vi "Read_EPICS_Client_PVs(DataSocket)DBL_20160318.vi"(7 "error in (no error)":errorcluster, 10 "PV name":string="SR-RF2-H2O-VBL:HeatLoad-SBP-HOM") -> (0 "error out 2":errorcluster, 2 "Value(String)":string, 3 "Value":dbl=588.4805608779573, 4 "quality":u64)   [LabVIEW 2013]
panel:
  out "values":T1
  out "found":bool
  out "replaced":bool
  out "variant out":variant
  out "data 3":bool
  out "Value 2":dbl=588.4805608779573
  out "data 2":string
  out "string":i16[](array[numeric])
  out "data string 4":string
  out "type string 2":i16[](array[numeric])
  out "data string 3":string
  out "data":variant
  in  "stop":bool
  out "loop":i32
  # "有@表示為數字"
  # "4\n10"
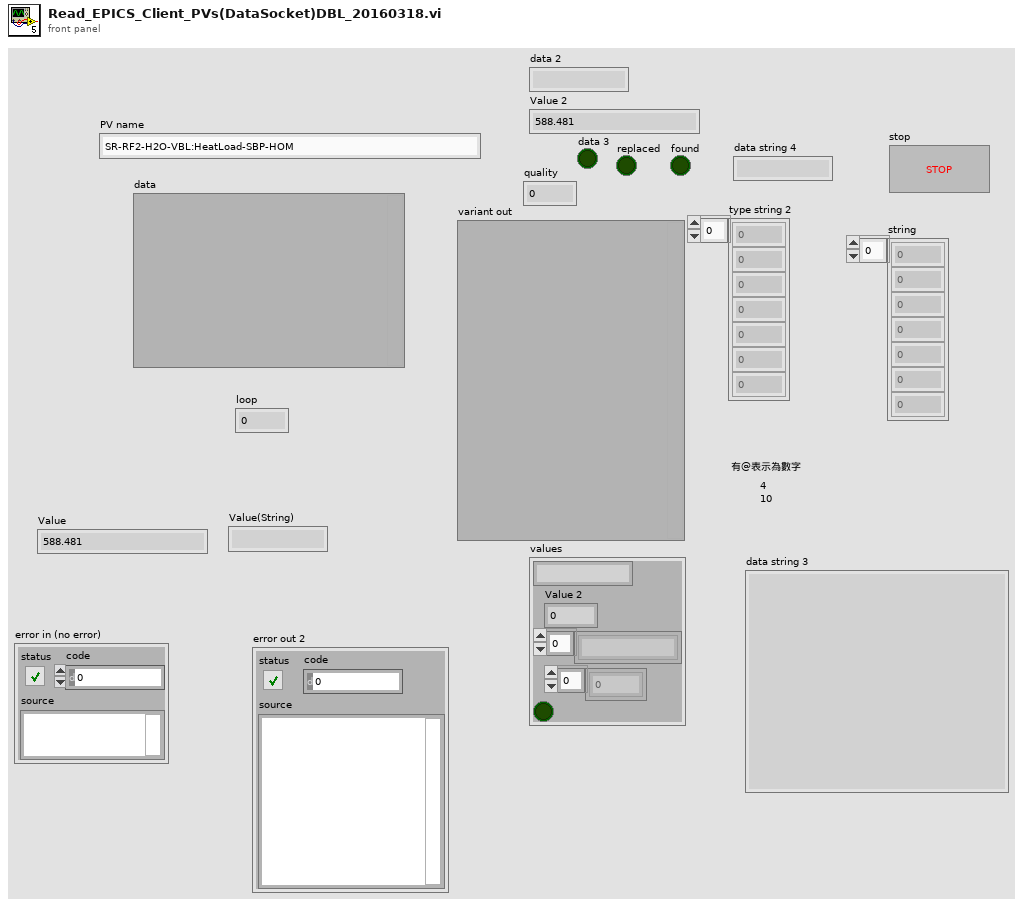
[diagram p1: front panel]
types:
  T1 = cluster{string, "Value 2":dbl, string[], dbl[], bool}
  T2 = enum16{"Read", "Write", "ReadWrite", "BufferedRead", "BufferedReadWrite"}
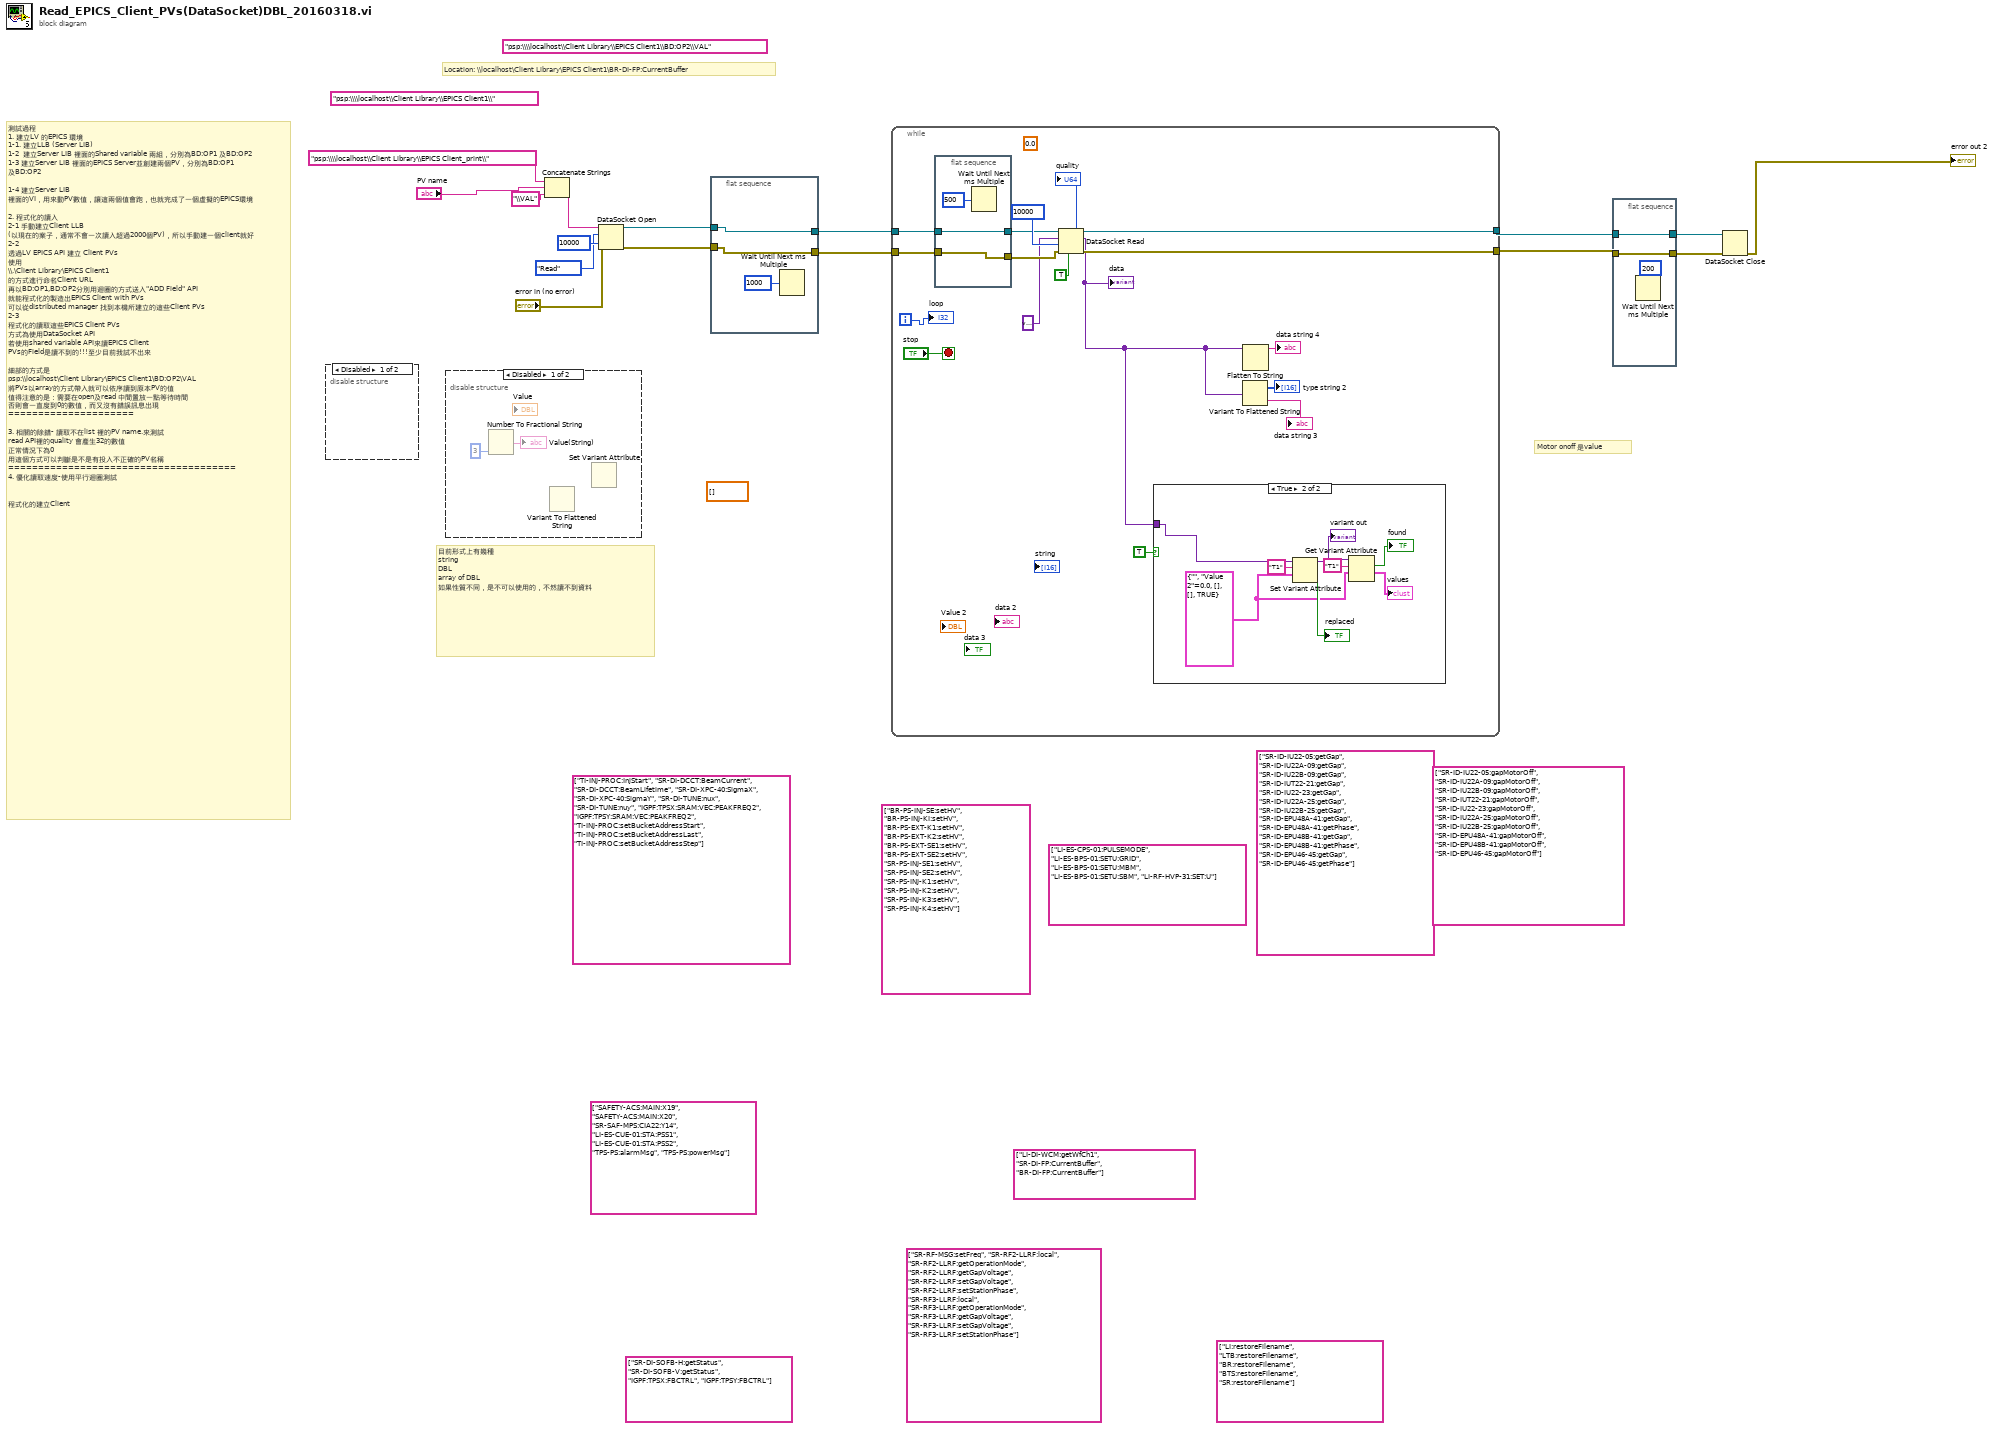
[diagram p0: block diagram]
diagram:
  (unwired) dbl[] []
  (unwired) string[] ["LI:restoreFilename", "LTB:restoreFilename", "BR:restoreFilename", "BTS:restoreFilename", "SR:restoreFilename"]
  (unwired) string[] ["SR-RF-MSG:setFreq", "SR-RF2-LLRF:local", "SR-RF2-LLRF:getOperationMode", "SR-RF2-LLRF:getGapVoltage", "SR-RF2-LLRF:setGapVoltage", "SR-RF2-LLRF:setStationPhase", "SR-RF3-LLRF:local", "SR-RF3-LLRF:getOperationMode", "SR-RF3-LLRF:getGapVoltage", "SR-RF3-LLRF:setGapVoltage", "SR-RF3-LLRF:setStationPhase"]
  (unwired) string[] ["SR-DI-SOFB-H:getStatus", "SR-DI-SOFB-V:getStatus", "IGPF:TPSX:FBCTRL", "IGPF:TPSY:FBCTRL"]
  (unwired) string[] ["LI-DI-WCM:getWfCh1", "SR-DI-FP:CurrentBuffer", "BR-DI-FP:CurrentBuffer"]
  (unwired) string[] ["SAFETY-ACS:MAIN:X19", "SAFETY-ACS:MAIN:X20", "SR-SAF-MPS:CIA22:Y14", "LI-ES-CUE-01:STA:PSS1", "LI-ES-CUE-01:STA:PSS2", "TPS-PS:alarmMsg", "TPS-PS:powerMsg"]
  (unwired) string[] ["SR-ID-IU22-05:gapMotorOff", "SR-ID-IU22A-09:gapMotorOff", "SR-ID-IU22B-09:gapMotorOff", "SR-ID-IUT22-21:gapMotorOff", "SR-ID-IU22-23:gapMotorOff", "SR-ID-IU22A-25:gapMotorOff", "SR-ID-IU22B-25:gapMotorOff", "SR-ID-EPU48A-41:gapMotorOff", "SR-ID-EPU48B-41:gapMotorOff", "SR-ID-EPU46-45:gapMotorOff"]
  (unwired) string[] ["SR-ID-IU22-05:getGap", "SR-ID-IU22A-09:getGap", "SR-ID-IU22B-09:getGap", "SR-ID-IUT22-21:getGap", "SR-ID-IU22-23:getGap", "SR-ID-IU22A-25:getGap", "SR-ID-IU22B-25:getGap", "SR-ID-EPU48A-41:getGap", "SR-ID-EPU48A-41:getPhase", "SR-ID-EPU48B-41:getGap", "SR-ID-EPU48B-41:getPhase", "SR-ID-EPU46-45:getGap", "SR-ID-EPU46-45:getPhase"]
  (unwired) string[] ["LI-ES-CPS-01:PULSEMODE", "LI-ES-BPS-01:SETU:GRID", "LI-ES-BPS-01:SETU:MBM", "LI-ES-BPS-01:SETU:SBM", "LI-RF-HVP-31:SET:U"]
  (unwired) string[] ["BR-PS-INJ-SE:setHV", "BR-PS-INJ-KI:setHV", "BR-PS-EXT-K1:setHV", "BR-PS-EXT-K2:setHV", "BR-PS-EXT-SE1:setHV", "BR-PS-EXT-SE2:setHV", "SR-PS-INJ-SE1:setHV", "SR-PS-INJ-SE2:setHV", "SR-PS-INJ-K1:setHV", "SR-PS-INJ-K2:setHV", "SR-PS-INJ-K3:setHV", "SR-PS-INJ-K4:setHV"]
  (unwired) string[] ["TI-INJ-PROC:InjStart", "SR-DI-DCCT:BeamCurrent", "SR-DI-DCCT:BeamLifetime", "SR-DI-XPC-40:SigmaX", "SR-DI-XPC-40:SigmaY", "SR-DI-TUNE:nux", "SR-DI-TUNE:nuy", "IGPF:TPSX:SRAM:VEC:PEAKFREQ2", "IGPF:TPSY:SRAM:VEC:PEAKFREQ2", "TI-INJ-PROC:setBucketAddressStart", "TI-INJ-PROC:setBucketAddressLast", "TI-INJ-PROC:setBucketAddressStep"]
  (unwired) "psp:\\\\localhost\\Client Library\\EPICS Client1\\" ("URL 2")
  (unwired) "psp:\\\\localhost\\Client Library\\EPICS Client1\\BD:OP2\\VAL" ("URL 2")
  # "Motor onoff 是value"
  # "目前形式上有幾種\nstring\nDBL\narray of DBL\n如果性質不同，是不可以使用的，不然讀不到資料"
  # "Location: \\\\localhost\\Client Library\\EPICS Client1\\BR-DI-FP:CurrentBuffer"
  # "測試過程\n1. 建立LV 的EPICS 環境\n1-1. 建立LLB (Server LIB) \n1-2  建立Server LIB 裡面的Shared variable 兩組，分別為BD:OP1 及BD:OP2\n1-3 建立Server LIB 裡面的EPICS Server並創建兩個PV，分別為BD:OP1 及BD:OP2\n\n1-4 建立Server LIB 裡面的VI，用來動PV數值，讓這兩個值會跑，也就完成了一個虛擬的EPICS環境\n\n2. 程式化的讀入\n2-1 手動建立Client LLB (以現在的案子，通常不會一次讀入超過2000個PV)，所以手動建一個client就好\n2-2\n透過LV EPICS API 建立 Client PVs\n使用\n\\\\.\\Client Library\\EPICS Client1\n的方式進行命名Client URL\n再以BD:OP1,BD:OP2分別用迴圈的方式送入\"ADD Field\" API\n就能程式化的製造出EPICS Client with PVs\n可以從distributed manager 找到本機所建立的這些Client PVs\n2-3\n程式化的讀取這些EPICS Client PVs\n方式為使用DataSocket API\n若使用shared variable API來讀EPICS Client PVs的Field是讀不到的!!!至少目前我試不出來\n\n細部的方式是\npsp:\\\\localhost\\Client Library\\EPICS Client1\\BD:OP2\\VAL\n將PVs以array的方式帶入就可以依序讀到原本PV的值\n值得注意的是：需要在open及read 中間置放一點等待時間\n否則會一直度到0的數值，而又沒有錯誤訊息出現\n=====================\n\n3. 相關的除錯- 讀取不在list 裡的PV name.來測試\nread API裡的quality 會產生32的數值\n正常情況下為0\n用這個方式可以判斷是不是有投入不正確的PV名稱\n======================================\n4. 優化讀取速度-使用平行迴圈測試\n\n\n程式化的建立Client"
  n1 = disable-structure shown="Disabled" {
    frame Disabled {
    }
    frame Enabled {
    }
  }
  n2 = disable-structure shown="Disabled" {
    frame Disabled {
      n3 = Number To Fractional String(precision (6)=i16 3) -> (F-format string=→"Value(String)":string)  [unwired: 3 in]
      n4 = Variant To Flattened String() -> ()  [unwired: 1 in, 2 out]
      n5 = Set Variant Attribute() -> ()  [unwired: 4 in, 3 out]
    }
    frame Enabled {
    }
  }
  n6 = Concatenate Strings("psp:\\\\localhost\\Client Library\\EPICS Client_print\\" ("URL 2"), "PV name", "\\VAL" ("URL 2")) -> (w5:string)
  n7 = DataSocket Open(8:"error in (no error)", 9:10000 ("ms timeout (10000)"), 10:T2."Read" ("mode"), 11:w5) -> (0:w3:errorcluster, 3:w4:refnum<k13>)
  n8 = flat-sequence {
    tunnel: w4 -> [w20]
    tunnel: w3 -> [w21]
    tunnel: [w21] -> w2
    tunnel: [w20] -> w1
    frame #0 {
      n9 = Wait Until Next ms Multiple(millisecond multiple=u32 1000) -> ()  [unwired: 1 out]
    }
  }
  n10 = while {
    tunnel: [w37] -> w16
    tunnel: [w36] -> w15
    tunnel: w1 -> [w33]
    tunnel: w2 -> [w30]
    i -> [w28]
    stop <- "stop" stop-if-true
    (unwired) 0.0
    n11 = flat-sequence {
      tunnel: w33 -> [w48]
      tunnel: [w48] -> w32
      tunnel: [w47] -> w31
      tunnel: w30 -> [w47]
      frame #0 {
        n12 = Wait Until Next ms Multiple(millisecond multiple=u32 500) -> ()  [unwired: 1 out]
      }
    }
    n13 = DataSocket Read(6:TRUE ("wait for updated value (T)"), 8:w31, 9:10000 ("ms timeout (10000)"), 10:variant ("type (Variant)"), 11:w32) -> (0:w37:errorcluster, 2:w22:variant, 3:w36:refnum<k13>, 5:→"quality":u64)  [unwired: 3 out]
    "data" <- w22
    n14 = case shown="True" TRUE {
      tunnel: w22 -> [_ w46]
      frame False {
      }
      frame True {
        w41 = T1 {"", "Value 2"=0.0, [], [], TRUE} ("value")
        n15 = Set Variant Attribute(Variant=w46, name="T1", value=w41) -> (Variant out=w44:variant, replaced=→"replaced":bool)  [unwired: 1 in, 1 out]
        "variant out" <- w44
        n16 = Get Variant Attribute(Variant=w44, name="T1", default value (empty Variant)=w41) -> (found=→"found":bool, value=→"values":T1)  [unwired: 1 in, 2 out]
      }
    }
    n17 = Variant To Flattened String(Variant=w22) -> (data string=→"data string 3":string, 1:→"type string 2":i16[])
    n18 = Flatten To String(anything=w22) -> (data string=→"data string 4":string)  [unwired: 3 in, 2 out]
    "loop" <- w28
  }
  n19 = flat-sequence {
    tunnel: w15 -> [w50]
    tunnel: w16 -> [w51]
    tunnel: [w51] -> w14
    tunnel: [w50] -> w13
    frame #0 {
      n20 = Wait Until Next ms Multiple(millisecond multiple=u32 200) -> ()  [unwired: 1 out]
    }
  }
  n21 = DataSocket Close(8:w14, 11:w13) -> (0:→"error out 2":errorcluster)  [unwired: 1 in, 1 out]
